vi "test FPGA UDVs.vi"(8 "error in (no error)":errorcluster, 11 "TestCase in":refnum<class "cRIO System Tests.lvclass">) -> (0 "error out":errorcluster, 3 "TestCase out":refnum<class "cRIO System Tests.lvclass">)   [LabVIEW 2019, in "cRIO System Tests.lvclass"]
uses:
  cRIO System Tests.lvclass
  C:/Users/nitest/Desktop/Git 2019/niveristand-custom-device-testing-tools/VeriStandTestCase/VeriStandTestCase.lvclass
  <vilib>/numeric/Random Number (Range) U64.vi
  <vilib>/numeric/Random Number (Range) I64.vi
  <vilib>/numeric/sub_Random U32.vi
  <vilib>/addons/_JKI Toolkits/VI Tester/TestCase.llb/TestCase.lvclass
  niveristand-custom-device-testing-tools/VeriStandTestCase/VeriStandTestCase.lvclass
  C:/Program Files (x86)/National Instruments/LabVIEW 2019/vi.lib/addons/_JKI Toolkits/VI Tester/TestCase.llb/TestCase.lvclass
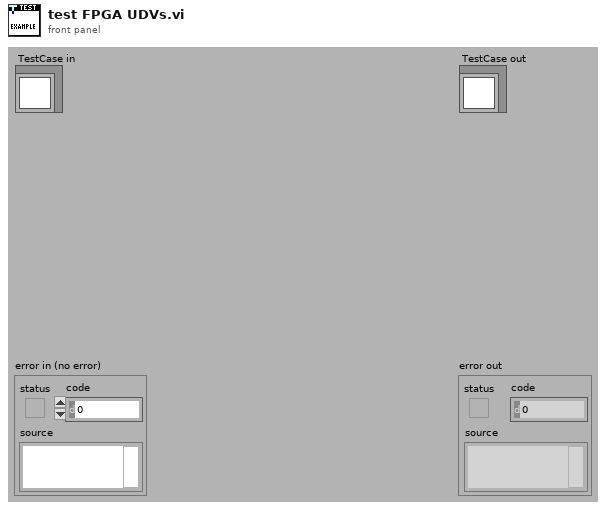
[diagram p1: front panel]
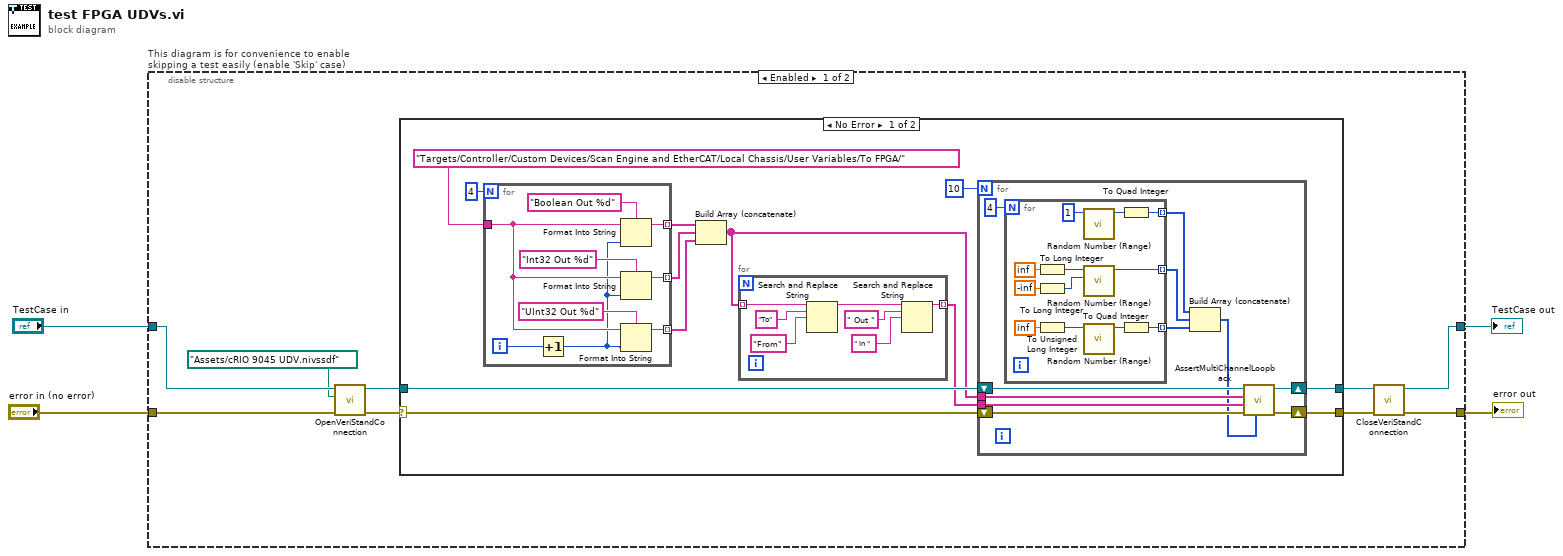
[diagram p0: block diagram]
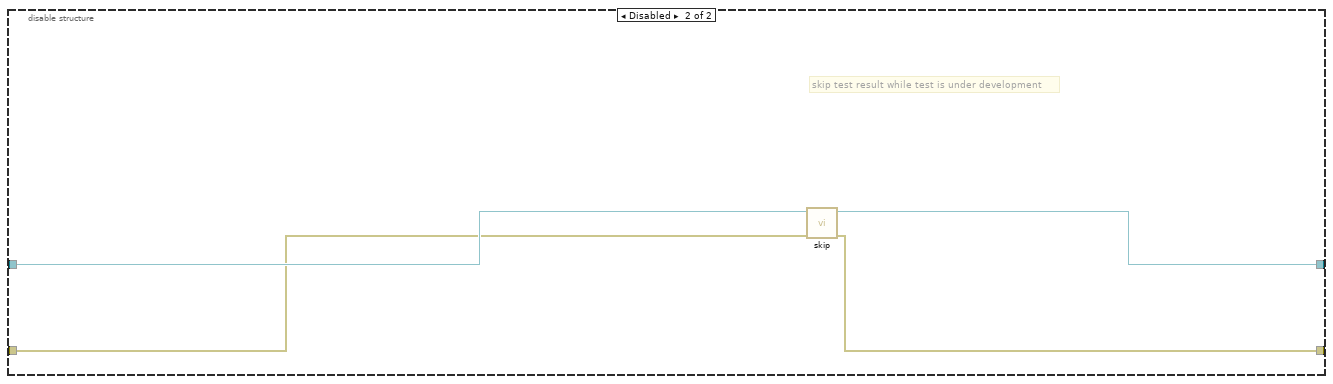
[diagram p3: hidden frame]
diagram:
  n1 = disable-structure "This diagram is for convenience to enable skipping a test easily (enable 'Skip' case)" shown="Enabled" {
    disable-tunnel: "TestCase in" -> [w10 w70]
    disable-tunnel: [w6 w68] -> w1
    disable-tunnel: [w8 w69] -> w3
    disable-tunnel: "error in (no error)" -> [w12 w67]
    frame Enabled {
      n2 = call-dynamic "OpenVeriStandConnection.vi"("error in (no error)"=w12, "System Definition File"=path "Assets/cRIO 9045 UDV.nivssdf", "VeriStand Test Case in"=w10) -> ("error out"=w13:errorcluster, "VeriStand Test Case out"=w11:refnum<class "cRIO System Tests.lvclass">)  [unwired: 6 in, 1 out]
      n3 = case shown="No Error" w13 {
        selector: w13 -> [w21 w66]
        tunnel: [w20 w66] -> w9
        tunnel: [w22 w65] -> w7
        tunnel: w11 -> [w23 w65]
        frame No Error {
          n4 = for {
            N: 4 -> [_]
            tunnel: "Targets/Controller/Custom Devices/Scan Engine and EtherCAT/Local Chassis/User Variables/To FPGA/" -> [w58]
            tunnel: [w63] -> w16 mode=indexing
            tunnel: [w61] -> w17 mode=indexing
            tunnel: [w57] -> w18 mode=indexing
            i -> [w59]
            n5 = Increment(x=w59) -> (x+1=w56:i32)
            n6 = Format Into String(format string="Boolean Out %d", initial string=w58, w56) -> (resulting string=w63:string)  [unwired: 1 in, 1 out]
            n7 = Format Into String(format string="Int32 Out %d", initial string=w58, w56) -> (resulting string=w61:string)  [unwired: 1 in, 1 out]
            n8 = Format Into String(format string="UInt32 Out %d", initial string=w58, w56) -> (resulting string=w57:string)  [unwired: 1 in, 1 out]
          }
          n9 = Build Array (concatenate)(w16, w17, w18) -> (w15:string[])
          n10 = for {
            tunnel: w15 -> [w55] mode=indexing
            tunnel: [w49] -> w14 mode=indexing
            n11 = Search and Replace String(input string=w55, search string="To", replace string="From" ("search string")) -> (result string=w50:string)  [unwired: 5 in, 3 out]
            n12 = Search and Replace String(input string=w50, search string=" Out ", replace string=" In " ("search string")) -> (result string=w49:string)  [unwired: 5 in, 3 out]
          }
          n13 = for {
            N: 10 -> [_]
            tunnel: w15 -> [w32]
            tunnel: w14 -> [w31]
            shift-right: [w35] -> w22
            shift-left: w23 -> [w36]
            shift-right: [w33] -> w20
            shift-left: w21 -> [w34]
            n14 = for {
              N: 4 -> [_]
              tunnel: [w41] -> w26 mode=indexing
              tunnel: [w40] -> w29 mode=indexing
              tunnel: [w45] -> w27 mode=indexing
              n15 = To Long Integer(number=inf) -> (32bit integer=w39:i32)
              n16 = To Long Integer(number=-inf) -> (32bit integer=w38:i32)
              n17 = To Unsigned Long Integer(number=inf) -> (unsigned 32bit integer=w37:u32)
              n18 = call-poly <vilib>:"Random Number (Range).vi"("upper bound (100)"=u64 1) -> ("number"=w48:u64)  [unwired: 10 in]
              n19 = call-poly <vilib>:"Random Number (Range).vi"("lower bound (-100)"=w38, "upper bound (100)"=w39) -> ("number"=w45:i64)  [unwired: 9 in]
              n20 = call-poly <vilib>:"Random Number (Range).vi"("upper bound (100)"=w37) -> ("number"=w46:u64)  [unwired: 10 in]
              n21 = To Quad Integer(1:w48) -> (0:w41:i64)
              n22 = To Quad Integer(1:w46) -> (0:w40:i64)
            }
            n23 = Build Array (concatenate)(w26, w27, w29) -> (w28:i64[])
            n24 = call "AssertMultiChannelLoopback.vi"("Values"=w28, "error in (no error)"=w34, "Read Channels"=w31, "Write Channels"=w32, "VeriStand Test Case in"=w36) -> ("error out"=w33:errorcluster, "VeriStand Test Case out"=w35:refnum<class "cRIO System Tests.lvclass">)  [unwired: 5 in]
          }
        }
        frame Error {
        }
      }
      n25 = call-dynamic "CloseVeriStandConnection.vi"("error in (no error)"=w9, "VeriStand Test Case in"=w7) -> ("error out"=w8:errorcluster, "VeriStand Test Case out"=w6:refnum<class "cRIO System Tests.lvclass">)  [unwired: 8 in]
    }
    frame Disabled {
      # "skip test result while test is under development"
      n26 = call <vilib>:"skip.vi"("error in (no error)"=w67, "TestCase in"=w70) -> ("error out"=w69:errorcluster, "TestCase out"=w68:refnum<class "cRIO System Tests.lvclass">)  [unwired: 8 in]
    }
  }
  "error out" <- w3
  "TestCase out" <- w1
